vi "populateTelemetryFPGAData.vi"(8 "error in (no error)":errorcluster, 10 "Data":u64[](array[numeric]), 11 "Model in":refnum<class "Model.lvclass">) -> (0 "error out":errorcluster, 3 "Model out":refnum<class "Model.lvclass">)   [LabVIEW 2016, in "Model.lvclass"]
uses:
  Model.lvclass
  DataTypes/Topics/TelemetryFPGAData.ctl
  DataTypes/Topics/Parts/Timestamp.ctl
  Model.lvclass/Model.ctl
  Publisher/Publisher.lvclass/Publisher.ctl
  DataTypes/Topics/M1M3SupportTopics.lvlib
  Publisher/Publisher.lvclass
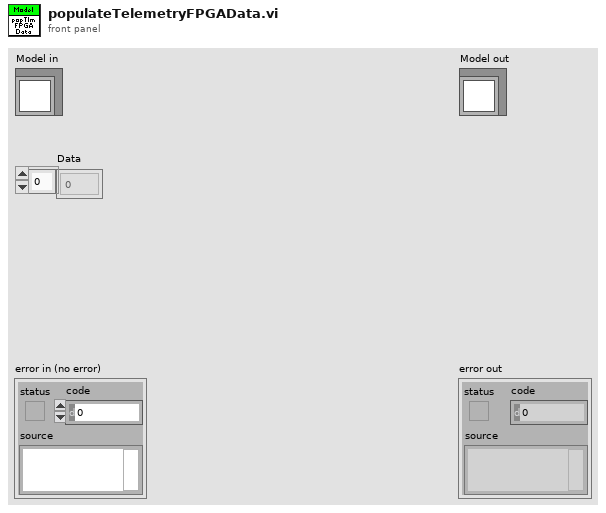
[diagram p1: front panel]
types:
  T1 = typedef "M1M3SupportTopics.lvlib/TelemetryFPGAData.ctl" = cluster{"Timestamp":T2, "ModbusSubnetATxInternalFIFOOverflow":bool, "ModbusSubnetAInvalidInstruction":bool, "ModbusSubnetAWaitForRxFrameTimeout":bool, "ModbusSubnetAStartBitError":bool, "ModbusSubnetAStopBitError":bool, "ModbusSubnetARxDataFIFOOverflow":bool, "ModbusSubnetATxByteCount":u32, "ModbusSubnetATxFrameCount":u32, "ModbusSubnetARxByteCount":u32, "ModbusSubnetARxFrameCount":u32, "ModbusSubnetBTxInternalFIFOOverflow":bool, "ModbusSubnetBInvalidInstruction":bool, "ModbusSubnetBWaitForRxFrameTimeout":bool, "ModbusSubnetBStartBitError":bool, "ModbusSubnetBStopBitError":bool, "ModbusSubnetBRxDataFIFOOverflow":bool, "ModbusSubnetBTxByteCount":u32, "ModbusSubnetBTxFrameCount":u32, "ModbusSubnetBRxByteCount":u32, "ModbusSubnetBRxFrameCount":u32, "ModbusSubnetCTxInternalFIFOOverflow":bool, "ModbusSubnetCInvalidInstruction":bool, "ModbusSubnetCWaitForRxFrameTimeout":bool, "ModbusSubnetCStartBitError":bool, "ModbusSubnetCStopBitError":bool, "ModbusSubnetCRxDataFIFOOverflow":bool, "ModbusSubnetCTxByteCount":u32, "ModbusSubnetCTxFrameCount":u32, "ModbusSubnetCRxByteCount":u32, "ModbusSubnetCRxFrameCount":u32, "ModbusSubnetDTxInternalFIFOOverflow":bool, "ModbusSubnetDInvalidInstruction":bool, "ModbusSubnetDWaitForRxFrameTimeout":bool, "ModbusSubnetDStartBitError":bool, "ModbusSubnetDStopBitError":bool, "ModbusSubnetDRxDataFIFOOverflow":bool, "ModbusSubnetDTxByteCount":u32, "ModbusSubnetDTxFrameCount":u32, "ModbusSubnetDRxByteCount":u32, "ModbusSubnetDRxFrameCount":u32, "ModbusSubnetETxInternalFIFOOverflow":bool, "ModbusSubnetEInvalidInstruction":bool, "ModbusSubnetEWaitForRxFrameTimeout":bool, "ModbusSubnetEStartBitError":bool, "ModbusSubnetEStopBitError":bool, "ModbusSubnetERxDataFIFOOverflow":bool, "ModbusSubnetETxByteCount":u32, "ModbusSubnetETxFrameCount":u32, "ModbusSubnetERxByteCount":u32, "ModbusSubnetERxFrameCount":u32, "FPGATimestamp":dbl}
  T2 = typedef "M1M3SupportTopics.lvlib/Timestamp.ctl" = dbl
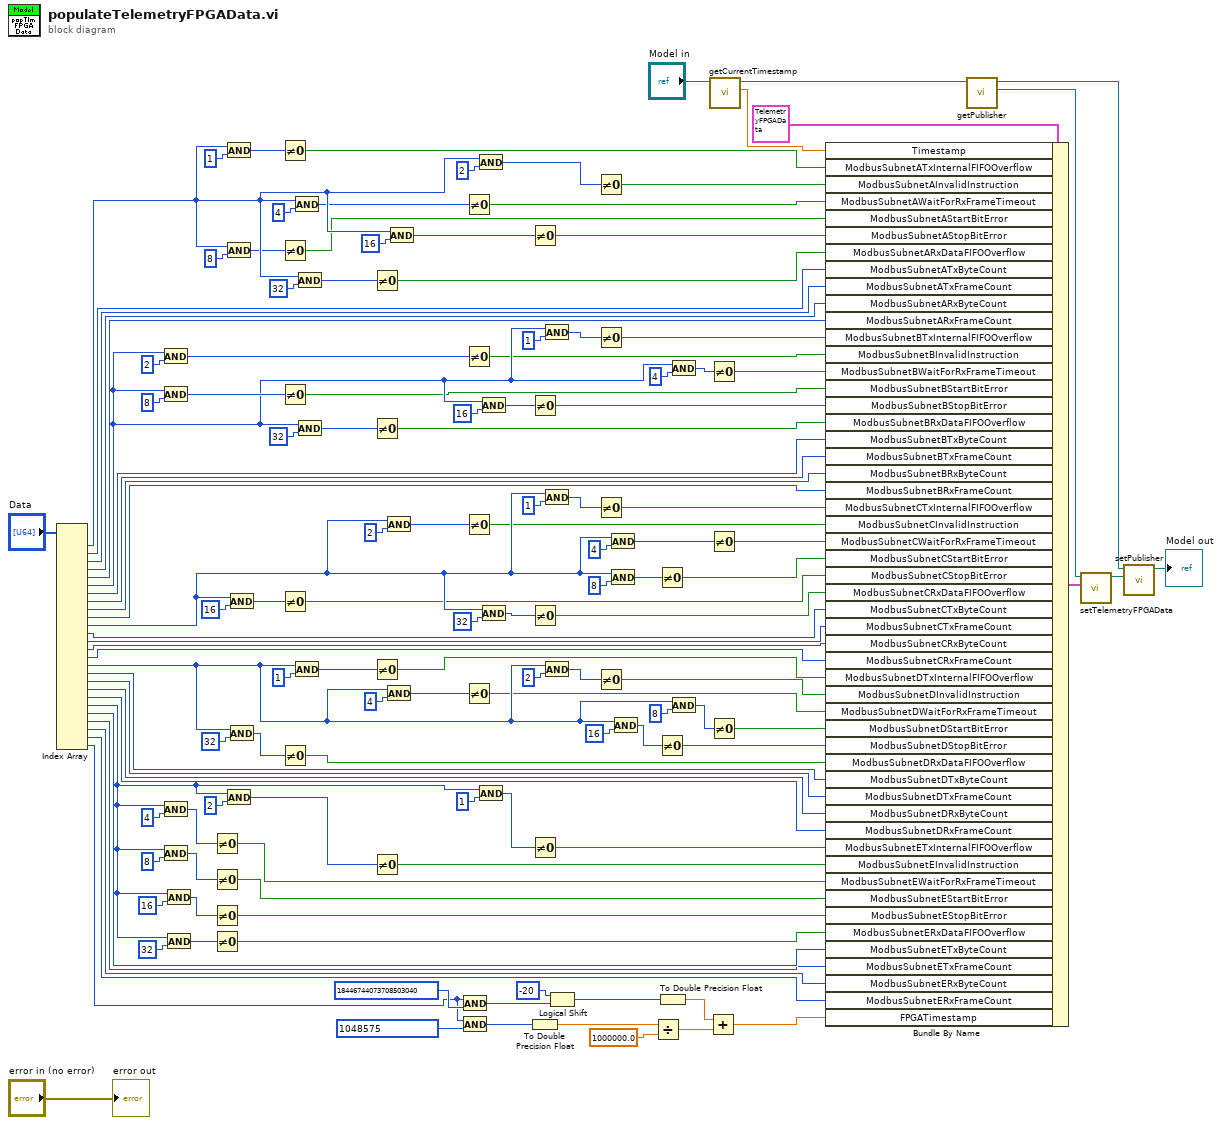
[diagram p0: block diagram]
diagram:
  n1 = Index Array(array="Data") -> (element #1=w126:u64, element #2=w135:u64, element #3=w134:u64, element #4=w133:u64, element #5=w132:u64, element #6=w96:u64, element #7=w131:u64, element #8=w130:u64, element #9=w129:u64, element #10=w128:u64, element #11=w77:u64, element #12=w70:u64, element #13=w69:u64, element #14=w68:u64, element #15=w67:u64, element #16=w54:u64, element #17=w47:u64, element #18=w46:u64, element #19=w45:u64, element #20=w44:u64, element #21=w31:u64, element #22=w24:u64, element #23=w23:u64, element #24=w22:u64, element #25=w21:u64, element #26=w1:u64)  [unwired: 26 in]
  n2 = And(x=w96, y=u32 2) -> (x .and. y?=w98:u64)
  n3 = And(x=w96, y=u32 8) -> (x .and. y?=w100:u64)
  n4 = And(x=w31, y=u32 4) -> (x .and. y?=w41:u64)
  n5 = And(x=w31, y=u32 8) -> (x .and. y?=w40:u64)
  n6 = And(x=w31, y=u32 16) -> (x .and. y?=w38:u64)
  n7 = And(x=w31, y=u32 32) -> (x .and. y?=w39:u64)
  n8 = Not Equal To 0?(x=w41) -> (x != 0?=w28:bool)
  n9 = Not Equal To 0?(x=w40) -> (x != 0?=w27:bool)
  n10 = Not Equal To 0?(x=w38) -> (x != 0?=w26:bool)
  n11 = Not Equal To 0?(x=w39) -> (x != 0?=w25:bool)
  n12 = And(x=w126, y=u32 1) -> (x .and. y?=w127:u64)
  n13 = And(x=w126, y=u32 8) -> (x .and. y?=w123:u64)
  n14 = And(x=w31, y=u32 2) -> (x .and. y?=w42:u64)
  n15 = And(x=w77, y=u32 16) -> (x .and. y?=w84:u64)
  n16 = And(x=w54, y=u32 32) -> (x .and. y?=w59:u64)
  n17 = Not Equal To 0?(x=w127) -> (x != 0?=w120:bool)
  n18 = Not Equal To 0?(x=w123) -> (x != 0?=w117:bool)
  n19 = Not Equal To 0?(x=w100) -> (x != 0?=w92:bool)
  n20 = Not Equal To 0?(x=w84) -> (x != 0?=w72:bool)
  n21 = Not Equal To 0?(x=w59) -> (x != 0?=w48:bool)
  n22 = And(x=w126, y=u32 4) -> (x .and. y?=w124:u64)
  n23 = And(x=w54, y=u32 1) -> (x .and. y?=w55:u64)
  n24 = And(x=w126, y=u32 32) -> (x .and. y?=w122:u64)
  n25 = And(x=w96, y=u32 32) -> (x .and. y?=w101:u64)
  n26 = Not Equal To 0?(x=w122) -> (x != 0?=w115:bool)
  n27 = Not Equal To 0?(x=w101) -> (x != 0?=w90:bool)
  n28 = Not Equal To 0?(x=w55) -> (x != 0?=w53:bool)
  n29 = Not Equal To 0?(x=w42) -> (x != 0?=w29:bool)
  n30 = And(x=w77, y=u32 2) -> (x .and. y?=w88:u64)
  n31 = And(x=w54, y=u32 4) -> (x .and. y?=w57:u64)
  n32 = And(x=w126, y=u32 16) -> (x .and. y?=w121:u64)
  n33 = And(x=w1, y=u64 18446744073708503040) -> (x .and. y?=w19:u64)
  n34 = And(x=w1, y=u64 1048575) -> (x .and. y?=w15:u64)
  n35 = Not Equal To 0?(x=w124) -> (x != 0?=w118:bool)
  n36 = Not Equal To 0?(x=w98) -> (x != 0?=w94:bool)
  n37 = Not Equal To 0?(x=w88) -> (x != 0?=w75:bool)
  n38 = Not Equal To 0?(x=w57) -> (x != 0?=w51:bool)
  n39 = And(x=w126, y=u32 2) -> (x .and. y?=w125:u64)
  n40 = And(x=w31, y=u32 1) -> (x .and. y?=w43:u64)
  n41 = And(x=w96, y=u32 16) -> (x .and. y?=w102:u64)
  n42 = And(x=w77, y=u32 32) -> (x .and. y?=w85:u64)
  n43 = Not Equal To 0?(x=w121) -> (x != 0?=w116:bool)
  n44 = Not Equal To 0?(x=w102) -> (x != 0?=w91:bool)
  n45 = Not Equal To 0?(x=w85) -> (x != 0?=w71:bool)
  n46 = Not Equal To 0?(x=w43) -> (x != 0?=w30:bool)
  n47 = To Double Precision Float(number=w15) -> (double precision float=w14:dbl)
  n48 = And(x=w96, y=u32 1) -> (x .and. y?=w97:u64)
  n49 = And(x=w77, y=u32 1) -> (x .and. y?=w89:u64)
  n50 = And(x=w54, y=u32 2) -> (x .and. y?=w56:u64)
  n51 = Logical Shift(y=i16 -20, x=w19) -> (x << y=w17:u64)
  n52 = Not Equal To 0?(x=w125) -> (x != 0?=w119:bool)
  n53 = Not Equal To 0?(x=w97) -> (x != 0?=w95:bool)
  n54 = Not Equal To 0?(x=w89) -> (x != 0?=w76:bool)
  n55 = Not Equal To 0?(x=w56) -> (x != 0?=w52:bool)
  n56 = And(x=w77, y=u32 4) -> (x .and. y?=w87:u64)
  n57 = And(x=w77, y=u32 8) -> (x .and. y?=w86:u64)
  n58 = And(x=w54, y=u32 16) -> (x .and. y?=w60:u64)
  n59 = Divide(x=w14, y=1000000.0) -> (x/y=w11:dbl)
  n60 = Not Equal To 0?(x=w86) -> (x != 0?=w73:bool)
  n61 = Not Equal To 0?(x=w60) -> (x != 0?=w49:bool)
  n62 = To Double Precision Float(number=w17) -> (double precision float=w12:dbl)
  n63 = And(x=w96, y=u32 4) -> (x .and. y?=w99:u64)
  n64 = And(x=w54, y=u32 8) -> (x .and. y?=w58:u64)
  n65 = Add(x=w12, y=w11) -> (x+y=w10:dbl)
  n66 = Not Equal To 0?(x=w99) -> (x != 0?=w93:bool)
  n67 = Not Equal To 0?(x=w87) -> (x != 0?=w74:bool)
  n68 = Not Equal To 0?(x=w58) -> (x != 0?=w50:bool)
  n69 = call "getCurrentTimestamp.vi"("Model in"="Model in") -> ("Timestamp"=w136:T2, "Model out"=w8:refnum<class "Model.lvclass">)  [unwired: 8 in, 1 out]
  n70 = Bundle By Name(cluster=T1 {"Timestamp"=0.0, "ModbusSubnetATxInternalFIFOOverflow"=FALSE, "ModbusSubnetAInvalidInstruction"=FALSE, "ModbusSubnetAWaitForRxFrameTimeout"=FALSE, "ModbusSubnetAStartBitError"=FALSE, "ModbusSubnetAStopBitError"=FALSE, "ModbusSubnetARxDataFIFOOverflow"=FALSE, "ModbusSubnetATxByteCount"=0, "ModbusSubnetATxFrameCount"=0, "ModbusSubnetARxByteCount"=0, "ModbusSubnetARxFrameCount"=0, "ModbusSubnetBTxInternalFIFOOverflow"=FALSE, "ModbusSubnetBInvalidInstruction"=FALSE, "ModbusSubnetBWaitForRxFrameTimeout"=FALSE, "ModbusSubnetBStartBitError"=FALSE, "ModbusSubnetBStopBitError"=FALSE, "ModbusSubnetBRxDataFIFOOverflow"=FALSE, "ModbusSubnetBTxByteCount"=0, "ModbusSubnetBTxFrameCount"=0, "ModbusSubnetBRxByteCount"=0, "ModbusSubnetBRxFrameCount"=0, "ModbusSubnetCTxInternalFIFOOverflow"=FALSE, "ModbusSubnetCInvalidInstruction"=FALSE, "ModbusSubnetCWaitForRxFrameTimeout"=FALSE, "ModbusSubnetCStartBitError"=FALSE, "ModbusSubnetCStopBitError"=FALSE, "ModbusSubnetCRxDataFIFOOverflow"=FALSE, "ModbusSubnetCTxByteCount"=0, "ModbusSubnetCTxFrameCount"=0, "ModbusSubnetCRxByteCount"=0, "ModbusSubnetCRxFrameCount"=0, "ModbusSubnetDTxInternalFIFOOverflow"=FALSE, "ModbusSubnetDInvalidInstruction"=FALSE, "ModbusSubnetDWaitForRxFrameTimeout"=FALSE, "ModbusSubnetDStartBitError"=FALSE, "ModbusSubnetDStopBitError"=FALSE, "ModbusSubnetDRxDataFIFOOverflow"=FALSE, "ModbusSubnetDTxByteCount"=0, "ModbusSubnetDTxFrameCount"=0, "ModbusSubnetDRxByteCount"=0, "ModbusSubnetDRxFrameCount"=0, "ModbusSubnetETxInternalFIFOOverflow"=FALSE, "ModbusSubnetEInvalidInstruction"=FALSE, "ModbusSubnetEWaitForRxFrameTimeout"=FALSE, "ModbusSubnetEStartBitError"=FALSE, "ModbusSubnetEStopBitError"=FALSE, "ModbusSubnetERxDataFIFOOverflow"=FALSE, "ModbusSubnetETxByteCount"=0, "ModbusSubnetETxFrameCount"=0, "ModbusSubnetERxByteCount"=0, "ModbusSubnetERxFrameCount"=0, "FPGATimestamp"=0.0} ("TelemetryFPGAData"), "Timestamp"=w136, "ModbusSubnetATxInternalFIFOOverflow"=w120, "ModbusSubnetAInvalidInstruction"=w119, "ModbusSubnetAWaitForRxFrameTimeout"=w118, "ModbusSubnetAStartBitError"=w117, "ModbusSubnetAStopBitError"=w116, "ModbusSubnetARxDataFIFOOverflow"=w115, "ModbusSubnetATxByteCount"=w135, "ModbusSubnetATxFrameCount"=w134, "ModbusSubnetARxByteCount"=w133, "ModbusSubnetARxFrameCount"=w132, "ModbusSubnetBTxInternalFIFOOverflow"=w95, "ModbusSubnetBInvalidInstruction"=w94, "ModbusSubnetBWaitForRxFrameTimeout"=w93, "ModbusSubnetBStartBitError"=w92, "ModbusSubnetBStopBitError"=w91, "ModbusSubnetBRxDataFIFOOverflow"=w90, "ModbusSubnetBTxByteCount"=w131, "ModbusSubnetBTxFrameCount"=w130, "ModbusSubnetBRxByteCount"=w129, "ModbusSubnetBRxFrameCount"=w128, "ModbusSubnetCTxInternalFIFOOverflow"=w76, "ModbusSubnetCInvalidInstruction"=w75, "ModbusSubnetCWaitForRxFrameTimeout"=w74, "ModbusSubnetCStartBitError"=w73, "ModbusSubnetCStopBitError"=w72, "ModbusSubnetCRxDataFIFOOverflow"=w71, "ModbusSubnetCTxByteCount"=w70, "ModbusSubnetCTxFrameCount"=w69, "ModbusSubnetCRxByteCount"=w68, "ModbusSubnetCRxFrameCount"=w67, "ModbusSubnetDTxInternalFIFOOverflow"=w53, "ModbusSubnetDInvalidInstruction"=w52, "ModbusSubnetDWaitForRxFrameTimeout"=w51, "ModbusSubnetDStartBitError"=w50, "ModbusSubnetDStopBitError"=w49, "ModbusSubnetDRxDataFIFOOverflow"=w48, "ModbusSubnetDTxByteCount"=w47, "ModbusSubnetDTxFrameCount"=w46, "ModbusSubnetDRxByteCount"=w45, "ModbusSubnetDRxFrameCount"=w44, "ModbusSubnetETxInternalFIFOOverflow"=w30, "ModbusSubnetEInvalidInstruction"=w29, "ModbusSubnetEWaitForRxFrameTimeout"=w28, "ModbusSubnetEStartBitError"=w27, "ModbusSubnetEStopBitError"=w26, "ModbusSubnetERxDataFIFOOverflow"=w25, "ModbusSubnetETxByteCount"=w24, "ModbusSubnetETxFrameCount"=w23, "ModbusSubnetERxByteCount"=w22, "ModbusSubnetERxFrameCount"=w21, "FPGATimestamp"=w10) -> (w6:T1)
  n71 = call "getPublisher.vi"("Model in"=w8) -> ("Publisher"=w7:refnum<class "Publisher.lvclass">, "Model out"=w4:refnum<class "Model.lvclass">)  [unwired: 9 in]
  n72 = call "setTelemetryFPGAData.vi"("TelemetryFPGAData"=w6, "Publisher in"=w7) -> ("Publisher out"=w5:refnum<class "Publisher.lvclass">)  [unwired: 9 in]
  n73 = call "setPublisher.vi"("Publisher"=w5, "Model in"=w4) -> ("Model out"=→"Model out":refnum<class "Model.lvclass">)  [unwired: 9 in]
  "error out" <- "error in (no error)"
